vi "Globals.vi"() -> ()   [LabVIEW 2017, in "nifxpmath_AddSub.xnode"]
uses:
  <vilib>/rvi/FXPMathLib/basic elements/FxpAddSub/XNode/nifxpmath_AddSub.xnode
panel:
  in  "TERM Ovfl NAME":string="overflow"
  in  "TERM LOADY NAME":string="use zero instead of x"
  in  "TERM LOADY ID":string="TERM_NLOADY"
  in  "TERM IsSub NAME":string="is sub?"
  in  "TERM IsSub ID":string="TERM_ISSUB"
  in  "TERM Bout NAME":string="borrow-out"
  in  "TERM Cout NAME":string="carry-out"
  in  "TERM CBout NAME":string="carry-out/inverted borrow-out"
  in  "TERM CBout ID":string="TERM_CBOUT"
  in  "TERM Bin NAME":string="borrow-in"
  in  "TERM Cin NAME":string="carry-in"
  in  "TERM CBin NAME":string="carry-in/inverted borrow-in"
  out "ADDSUB ICON":picture
  in  "TERM S NAME":string="s"
  in  "TERM Y NAME":string="y"
  in  "TERM X NAME":string="x"
  in  "TERM CBin ID":string="TERM_CBIN"
  in  "TERM S ID":string="TERM_S"
  in  "TERM Y ID":string="TERM_Y"
  in  "TERM X ID":string="TERM_X"
  out "SUB ICON":picture
  out "ADD ICON":picture
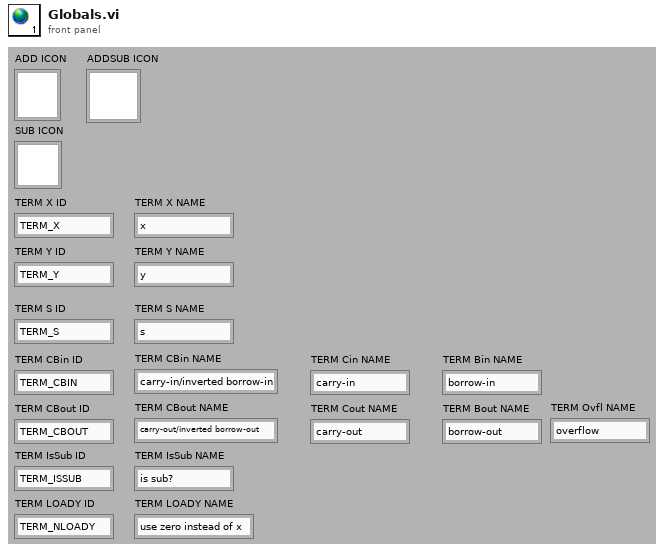
[diagram p1: front panel]
diagram:
